vi "Wave1D_Init Data_BC_Impl.vi"(9 "delta x":dbl, 10 "ks":dbl, 11 "Boundary Condition":cluster{"type":T1, "Value":dbl[]} {"type" items=["Dirichlet", "Neumann"]}) -> (3 "BC":cluster{"type":T1, "Value":dbl[]} {"type" items=["Dirichlet", "Neumann"]})   [LabVIEW 2017, in "NI_PDE.lvlib"]
uses:
  <vilib>/gmath/NI_PDE.lvlib
  <vilib>/gmath/pde.llb/Common/PDE_BC Type.ctl
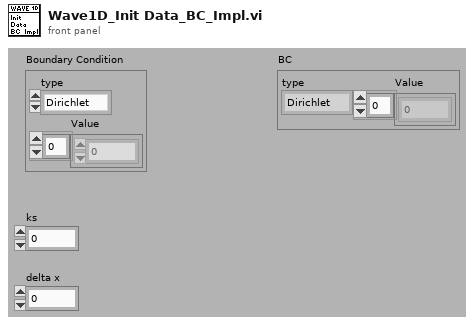
[diagram p1: front panel]
types:
  T1 = typedef "NI_PDE.lvlib/PDE_BC Type.ctl" = i32
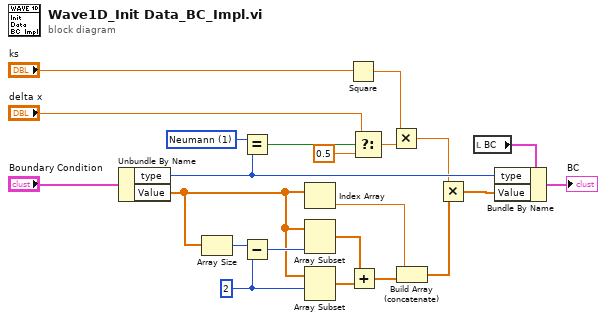
[diagram p0: block diagram]
diagram:
  w18 = T1 1 items=["Dirichlet", "Neumann"] ("x")
  w8 = 2 ("index")
  n1 = Unbundle By Name("Boundary Condition") -> ("type"=w19:T1, "Value"=w2:dbl[])
  n2 = Array Size(array=w2) -> (size(s)=w9:i32)
  n3 = Equal?(x=w18, y=w19) -> (x = y?=w17:bool)
  n4 = Subtract(x=w9, y=w8) -> (x-y=w7:i32)
  n5 = Index Array(array=w2) -> (element=w1:dbl)  [unwired: 1 in]
  n6 = Array Subset(array=w2, length=w7) -> (w6:dbl[])  [unwired: 1 in]
  n7 = Array Subset(array=w2, index=w8) -> (w5:dbl[])  [unwired: 1 in]
  n8 = Square(x="ks") -> (x^2=w12:dbl)
  n9 = Add(x=w6, y=w5) -> (x+y=w4:dbl[])
  n10 = Select(t="delta x", s=w17, f=0.5) -> (s? t:f=w14:dbl)
  n11 = Multiply(x=w12, y=w14) -> (x*y=w11:dbl)
  n12 = Build Array (concatenate)(w1, w4) -> (w3:dbl[])
  n13 = Multiply(x=w11, y=w3) -> (x*y=w10:dbl[])
  n14 = local read "BC"() -> (w21:cluster{"type":T1, "Value":dbl[]})
  n15 = Bundle By Name(cluster=w21, "type"=w19, "Value"=w10) -> (→"BC":cluster{"type":T1, "Value":dbl[]})
